vi "add values.vi"(4 "name":string, 5 "index string":string, 6 "is attribute?":bool, 7 "is array element?":bool, 8 "error in (no error)":errorcluster, 9 "Item Indent":i32, 10 "Variant":variant, 11 "Items in":T1(array[cluster])) -> (0 "error out":errorcluster, 3 "Items out":T1(array[cluster]))   [LabVIEW 2016]
uses:
  get unit string.vi
  <vilib>/Utility/Data Type/Get Numeric Information.vi
  <vilib>/Utility/Data Type/Get Cluster Information.vi
  <vilib>/Utility/LVClass/Get LV Class Name.vi
  <vilib>/Utility/Data Type/Get Fixed-Point Information.vi
  <vilib>/Utility/Data Type/Get Refnum Information.vi
  <vilib>/Utility/Data Type/NI_Data Type.lvlib
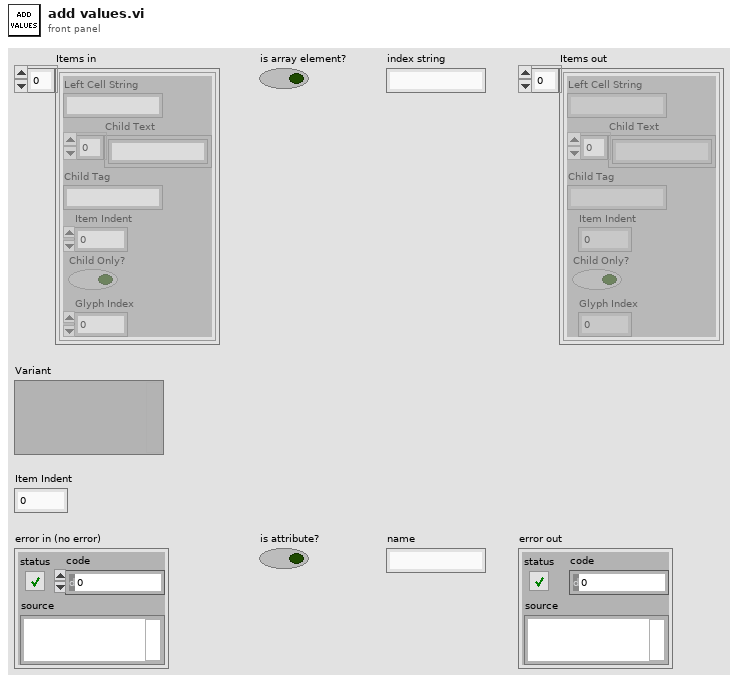
[diagram p1: front panel]
types:
  T1 = cluster{"Left Cell String":string, "Child Text":string[], "Child Tag":string, "Item Indent":i32, "Child Only?":bool, "Glyph Index":i32}[]
  T2 = typedef "NI_Data Type.lvlib/Data Type.ctl" = enum8{"Invalid Type", "Void", "I8", "I16", "I32", "I64", "U8", "U16", "U32", "U64", "Single Float", "Double Float", "Extended Float", "Single Complex", "Double Complex", "Extended Complex", "Enum U8", "Enum U16", "Enum U32", "Enum U64", "Single Float With Unit", "Double Float With Unit", "Extended Float With Unit", "Single Complex with Unit", "Double Complex with Unit", "Extended Complex with Unit", "Boolean", "String", "Path", "Picture", "Tag", "Array", "Cluster", "Variant", "LV Variant", "Waveform", "Timestamp", "Digital Waveform", "Digital Data", "ExpressData", "Refnum", "External Data", "VI", "Poly VI", "LabVIEW Class Instance", "Fixed Point"}
  T3 = cluster{"Left Cell String":string, "Child Text":string[], "Child Tag":string, "Item Indent":i32, "Child Only?":bool, "Glyph Index":i32}
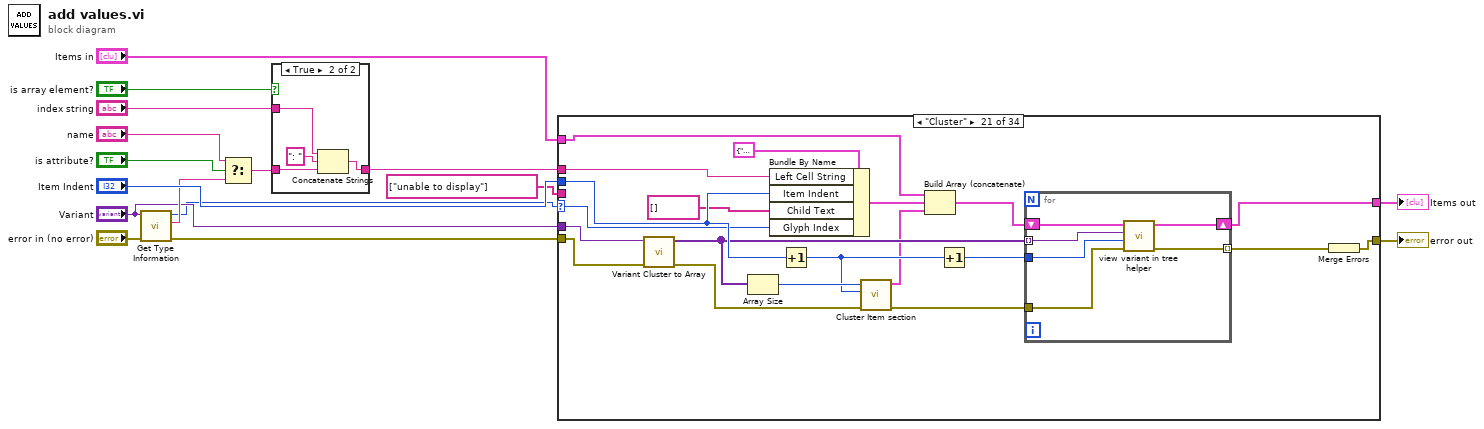
[diagram p0: block diagram]
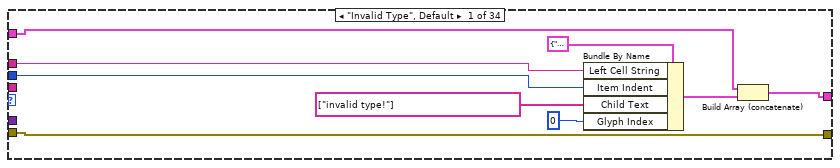
[diagram p3: hidden frame]
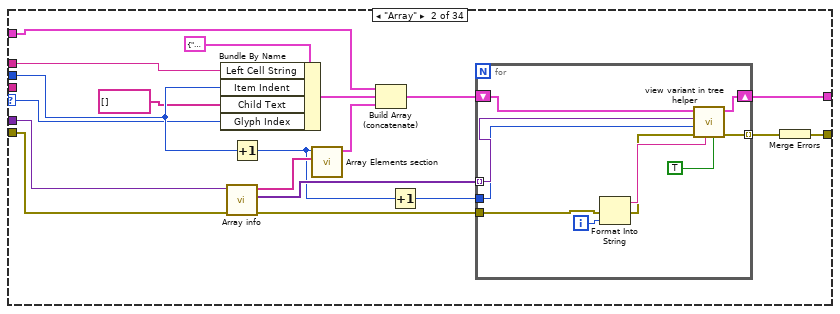
[diagram p4: hidden frame]
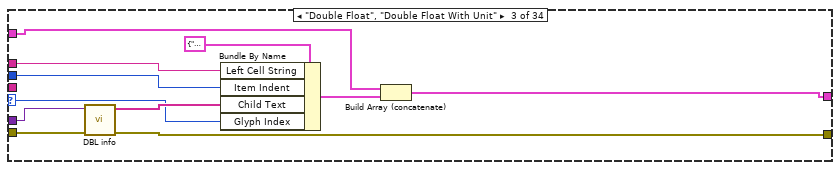
[diagram p5: hidden frame]
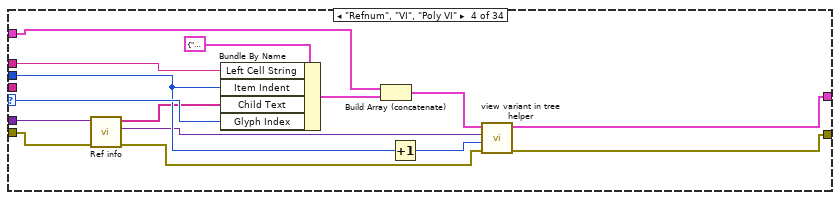
[diagram p6: hidden frame]
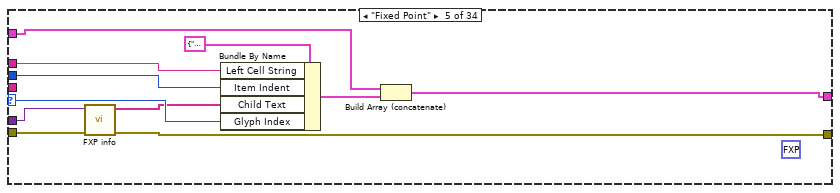
[diagram p7: hidden frame]
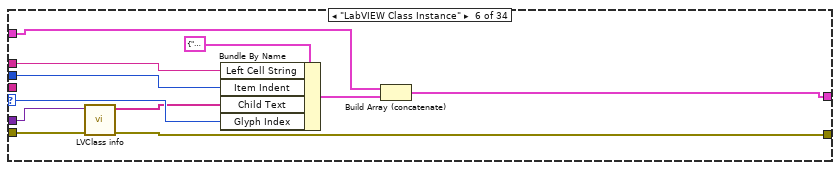
[diagram p8: hidden frame]
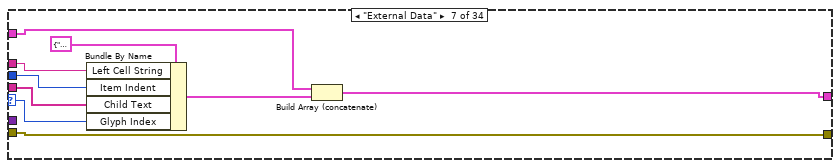
[diagram p9: hidden frame]
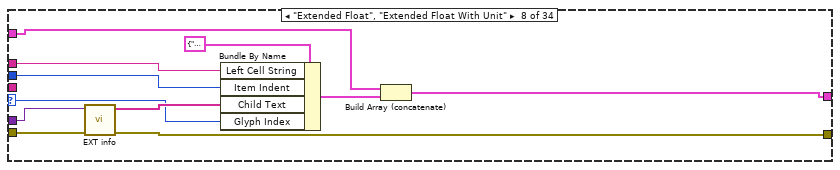
[diagram p10: hidden frame]
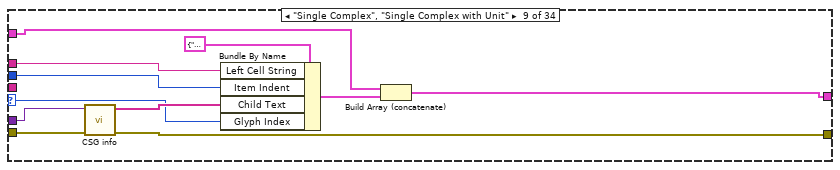
[diagram p11: hidden frame]
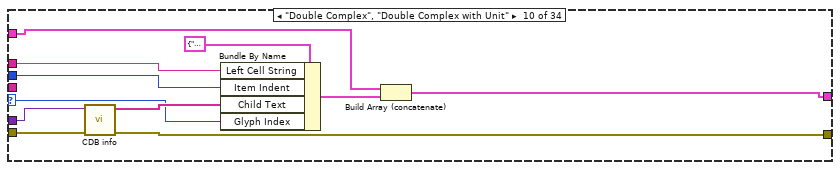
[diagram p12: hidden frame]
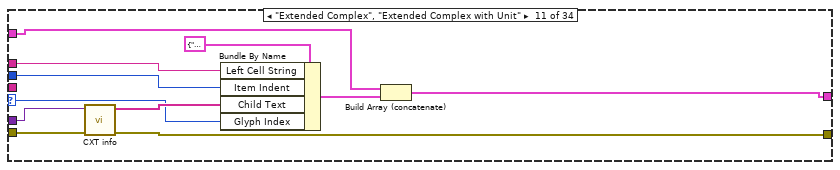
[diagram p13: hidden frame]
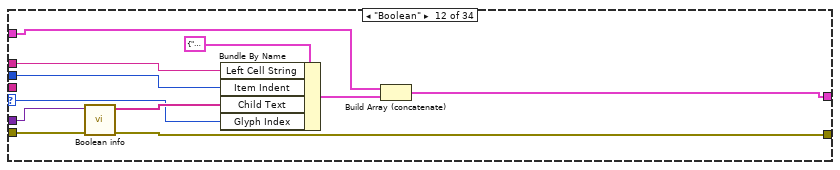
[diagram p14: hidden frame]
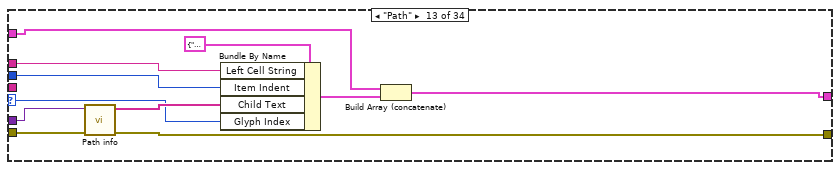
[diagram p15: hidden frame]
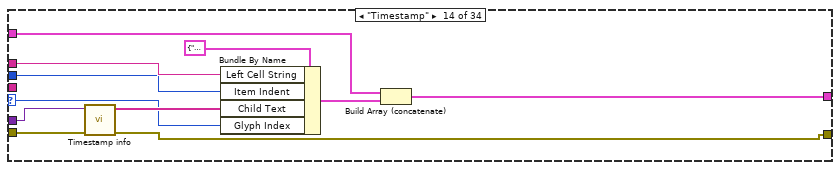
[diagram p16: hidden frame]
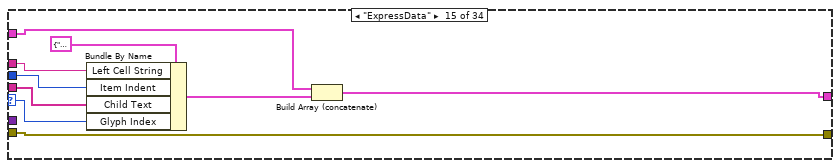
[diagram p17: hidden frame]
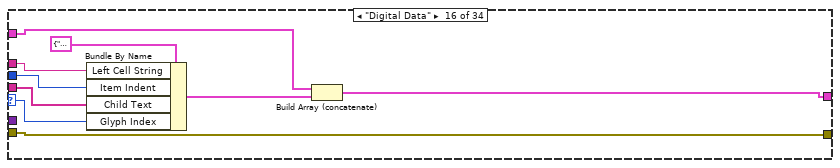
[diagram p18: hidden frame]
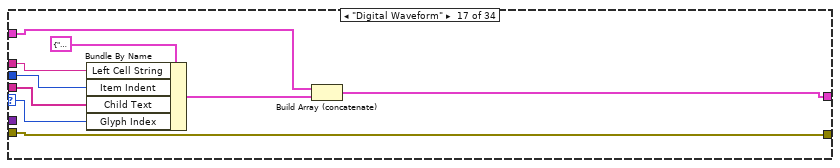
[diagram p19: hidden frame]
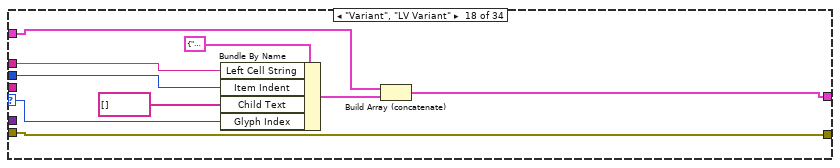
[diagram p20: hidden frame]
diagram:
  n1 = call <vilib>:"Get Type Information.vi"("error in (no error)"="error in (no error)", "Variant"="Variant") -> ("error out"=w15:errorcluster, "Name"=w7:string, "Type"=w1:T2)  [unwired: 5 in, 2 out]
  n2 = Select(t="name", s="is attribute?", f=w7) -> (s? t:f=w12:string)
  n3 = case shown="True" "is array element?" {
    tunnel: "index string" -> [_ w21]
    tunnel: w12 -> [w17 w19]
    tunnel: [w17 w18] -> w13
    frame False {
    }
    frame True {
      n4 = Concatenate Strings(w21, ": " ("string"), w19) -> (w18:string)
    }
  }
  n5 = case shown="\"Cluster\"" w1 {
    selector: w1 -> [_ w39 w64 w82 w90 w101 w110 w120 w131 w142 w153 w163 w174 w185 w195 w204 w213 w223 w232 w240 w257 w275 w284 w294 w305 w317 w327 w338 w349 w360 w371 w382 w393 w404]
    tunnel: "Items in" -> [w25 w46 w67 w80 w93 w104 w113 w123 w134 w145 w156 w166 w177 w188 w199 w208 w217 w227 w236 w244 w265 w279 w288 w297 w310 w321 w332 w343 w354 w365 w376 w387 w398 w409]
    tunnel: "Variant" -> [_ w49 w60 w81 w87 w98 _ w119 w129 w140 w151 w168 w179 w190 _ _ _ _ _ _ w258 _ _ w299 w307 w316 w329 w340 w351 w362 w373 w384 w395 w406]
    tunnel: w13 -> [w22 w40 w61 w84 w95 w106 w115 w126 w137 w148 w159 w170 w181 w192 w201 w210 w219 w228 w237 w246 w266 w281 w290 w301 w312 w323 w334 w345 w356 w367 w378 w389 w400 w411]
    tunnel: "Item Indent" -> [w28 w47 w69 w77 w94 w105 w114 w125 w136 w147 w158 w169 w180 w191 w200 w209 w218 w224 w233 w245 w261 w280 w289 w300 w311 w322 w333 w344 w355 w366 w377 w388 w399 w410]
    tunnel: [w23 w43 w65 w78 w91 w102 w111 w121 w132 w143 w154 w164 w175 w186 w197 w206 w215 w225 w234 w242 w262 w277 w286 w295 w308 w319 w330 w341 w352 w363 w374 w385 w396 w407] -> w5
    tunnel: string[] ["unable to display"] ("Child Text") -> [_ _ _ _ _ _ w108 _ _ _ _ _ _ _ w196 w205 w214 _ _ w241 _ w276 w285 _ _ _ _ _ _ _ _ _ _ _]
    tunnel: w15 -> [w30 w38 w63 w72 w89 w100 w109 w118 w130 w139 w152 w162 w173 w184 w194 w203 w212 w222 w231 w239 w256 w274 w283 w293 w304 w315 w326 w337 w348 w359 w370 w381 w392 w403]
    tunnel: [w30 w35 w62 w75 w88 w99 w109 w117 w128 w141 w150 w161 w172 w183 w194 w203 w212 w222 w231 w239 w252 w274 w283 w292 w303 w314 w325 w336 w347 w358 w369 w380 w391 w402] -> w16
    frame "Invalid Type", Default {
      n6 = Bundle By Name(cluster=T3 {"Left Cell String"="", "Child Text"=[], "Child Tag"="", "Item Indent"=0, "Child Only?"=FALSE, "Glyph Index"=0} ("Item"), "Left Cell String"=w22, "Item Indent"=w28, "Child Text"=string[] ["invalid type!"], "Glyph Index"=0) -> (w24:T3)
      n7 = Build Array (concatenate)(w25, w24) -> (w23:T1)
    }
    frame "Array" {
      n8 = Bundle By Name(cluster=T3 {"Left Cell String"="", "Child Text"=[], "Child Tag"="", "Item Indent"=0, "Child Only?"=FALSE, "Glyph Index"=0} ("Item"), "Left Cell String"=w40, "Item Indent"=w47, "Child Text"=string[] [], "Glyph Index"=w39) -> (w45:T3)
      n9 = call "Array info.vi"("error in (no error)"=w38, "Variant"=w49) -> ("error out"=w37:errorcluster, "elements"=w42:variant[], "child strings"=w41:string[])  [unwired: 7 in]
      n10 = Increment(x=w47) -> (x+1=w34:i32)
      n11 = call "Array Elements section.vi"("child strings"=w41, "indent"=w34) -> ("Array Elements section"=w33:T3)  [unwired: 9 in]
      n12 = Build Array (concatenate)(w46, w45, w33) -> (w44:T1)
      n13 = Increment(x=w34) -> (x+1=w31:i32)
      n14 = for {
        tunnel: w42 -> [w57] mode=indexing
        shift-right: [w58] -> w43
        shift-left: w44 -> [w59]
        tunnel: w31 -> [w56]
        tunnel: w37 -> [w52]
        tunnel: [w50] -> w36 mode=indexing
        i -> [w55]
        n15 = Format Into String(error in=w52, w55) -> (resulting string=w54:string, error out=w51:errorcluster)  [unwired: 2 in]
        n16 = call "view variant in tree helper.vi"("is array element?"=TRUE, "index string"=w54, "error in (no error)"=w51, "Item Indent"=w56, "Variant"=w57, "Items"=w59) -> ("error out"=w50:errorcluster, "Items out"=w58:T1)  [unwired: 4 in]
      }
      n17 = Merge Errors(w36) -> (w35:errorcluster)
    }
    frame "Double Float", "Double Float With Unit" {
      n18 = call "DBL info.vi"("error in (no error)"=w63, "Variant"=w60) -> ("error out"=w62:errorcluster, "child strings"=w68:string[])  [unwired: 8 in]
      n19 = Bundle By Name(cluster=T3 {"Left Cell String"="", "Child Text"=[], "Child Tag"="", "Item Indent"=0, "Child Only?"=FALSE, "Glyph Index"=0} ("Item"), "Left Cell String"=w61, "Item Indent"=w69, "Child Text"=w68, "Glyph Index"=w64) -> (w66:T3)
      n20 = Build Array (concatenate)(w67, w66) -> (w65:T1)
    }
    frame "Refnum", "VI", "Poly VI" {
      n21 = call "Ref info.vi"("error in (no error)"=w72, "Variant"=w81) -> ("error out"=w71:errorcluster, "refnum type"=w73:variant, "child strings"=w74:string[])  [unwired: 7 in]
      n22 = Bundle By Name(cluster=T3 {"Left Cell String"="", "Child Text"=[], "Child Tag"="", "Item Indent"=0, "Child Only?"=FALSE, "Glyph Index"=0} ("Item"), "Left Cell String"=w84, "Item Indent"=w77, "Child Text"=w74, "Glyph Index"=w82) -> (w83:T3)
      n23 = Build Array (concatenate)(w80, w83) -> (w79:T1)
      n24 = Increment(x=w77) -> (x+1=w76:i32)
      n25 = call "view variant in tree helper.vi"("error in (no error)"=w71, "Item Indent"=w76, "Variant"=w73, "Items"=w79) -> ("error out"=w75:errorcluster, "Items out"=w78:T1)  [unwired: 6 in]
    }
    frame "Fixed Point" {
      (unwired) fxp<+,1,1> 0.0
      n26 = call "FXP info.vi"("error in (no error)"=w89, "Variant"=w87) -> ("error out"=w88:errorcluster, "child strings"=w86:string[])  [unwired: 8 in]
      n27 = Bundle By Name(cluster=T3 {"Left Cell String"="", "Child Text"=[], "Child Tag"="", "Item Indent"=0, "Child Only?"=FALSE, "Glyph Index"=0} ("Item"), "Left Cell String"=w95, "Item Indent"=w94, "Child Text"=w86, "Glyph Index"=w90) -> (w92:T3)
      n28 = Build Array (concatenate)(w93, w92) -> (w91:T1)
    }
    frame "LabVIEW Class Instance" {
      n29 = call "LVClass info.vi"("error in (no error)"=w100, "Variant"=w98) -> ("error out"=w99:errorcluster, "child strings"=w97:string[])  [unwired: 8 in]
      n30 = Bundle By Name(cluster=T3 {"Left Cell String"="", "Child Text"=[], "Child Tag"="", "Item Indent"=0, "Child Only?"=FALSE, "Glyph Index"=0} ("Item"), "Left Cell String"=w106, "Item Indent"=w105, "Child Text"=w97, "Glyph Index"=w101) -> (w103:T3)
      n31 = Build Array (concatenate)(w104, w103) -> (w102:T1)
    }
    frame "External Data" {
      n32 = Bundle By Name(cluster=T3 {"Left Cell String"="", "Child Text"=[], "Child Tag"="", "Item Indent"=0, "Child Only?"=FALSE, "Glyph Index"=0} ("Item"), "Left Cell String"=w115, "Item Indent"=w114, "Child Text"=w108, "Glyph Index"=w110) -> (w112:T3)
      n33 = Build Array (concatenate)(w113, w112) -> (w111:T1)
    }
    frame "Extended Float", "Extended Float With Unit" {
      n34 = call "EXT info.vi"("error in (no error)"=w118, "Variant"=w119) -> ("error out"=w117:errorcluster, "child strings"=w124:string[])  [unwired: 8 in]
      n35 = Bundle By Name(cluster=T3 {"Left Cell String"="", "Child Text"=[], "Child Tag"="", "Item Indent"=0, "Child Only?"=FALSE, "Glyph Index"=0} ("Item"), "Left Cell String"=w126, "Item Indent"=w125, "Child Text"=w124, "Glyph Index"=w120) -> (w122:T3)
      n36 = Build Array (concatenate)(w123, w122) -> (w121:T1)
    }
    frame "Single Complex", "Single Complex with Unit" {
      n37 = call "CSG info.vi"("error in (no error)"=w130, "Variant"=w129) -> ("error out"=w128:errorcluster, "child strings"=w135:string[])  [unwired: 8 in]
      n38 = Bundle By Name(cluster=T3 {"Left Cell String"="", "Child Text"=[], "Child Tag"="", "Item Indent"=0, "Child Only?"=FALSE, "Glyph Index"=0} ("Item"), "Left Cell String"=w137, "Item Indent"=w136, "Child Text"=w135, "Glyph Index"=w131) -> (w133:T3)
      n39 = Build Array (concatenate)(w134, w133) -> (w132:T1)
    }
    frame "Double Complex", "Double Complex with Unit" {
      n40 = call "CDB info.vi"("error in (no error)"=w139, "Variant"=w140) -> ("error out"=w141:errorcluster, "child strings"=w146:string[])  [unwired: 8 in]
      n41 = Bundle By Name(cluster=T3 {"Left Cell String"="", "Child Text"=[], "Child Tag"="", "Item Indent"=0, "Child Only?"=FALSE, "Glyph Index"=0} ("Item"), "Left Cell String"=w148, "Item Indent"=w147, "Child Text"=w146, "Glyph Index"=w142) -> (w144:T3)
      n42 = Build Array (concatenate)(w145, w144) -> (w143:T1)
    }
    frame "Extended Complex", "Extended Complex with Unit" {
      n43 = call "CXT info.vi"("error in (no error)"=w152, "Variant"=w151) -> ("error out"=w150:errorcluster, "child strings"=w157:string[])  [unwired: 8 in]
      n44 = Bundle By Name(cluster=T3 {"Left Cell String"="", "Child Text"=[], "Child Tag"="", "Item Indent"=0, "Child Only?"=FALSE, "Glyph Index"=0} ("Item"), "Left Cell String"=w159, "Item Indent"=w158, "Child Text"=w157, "Glyph Index"=w153) -> (w155:T3)
      n45 = Build Array (concatenate)(w156, w155) -> (w154:T1)
    }
    frame "Boolean" {
      n46 = call "Boolean info.vi"("error in (no error)"=w162, "Variant"=w168) -> ("error out"=w161:errorcluster, "child strings"=w167:string[])  [unwired: 8 in]
      n47 = Bundle By Name(cluster=T3 {"Left Cell String"="", "Child Text"=[], "Child Tag"="", "Item Indent"=0, "Child Only?"=FALSE, "Glyph Index"=0} ("Item"), "Left Cell String"=w170, "Item Indent"=w169, "Child Text"=w167, "Glyph Index"=w163) -> (w165:T3)
      n48 = Build Array (concatenate)(w166, w165) -> (w164:T1)
    }
    frame "Path" {
      n49 = call "Path info.vi"("error in (no error)"=w173, "Variant"=w179) -> ("error out"=w172:errorcluster, "child strings"=w178:string[])  [unwired: 8 in]
      n50 = Bundle By Name(cluster=T3 {"Left Cell String"="", "Child Text"=[], "Child Tag"="", "Item Indent"=0, "Child Only?"=FALSE, "Glyph Index"=0} ("Item"), "Left Cell String"=w181, "Item Indent"=w180, "Child Text"=w178, "Glyph Index"=w174) -> (w176:T3)
      n51 = Build Array (concatenate)(w177, w176) -> (w175:T1)
    }
    frame "Timestamp" {
      n52 = call "Timestamp info.vi"("error in (no error)"=w184, "Variant"=w190) -> ("error out"=w183:errorcluster, "child strings"=w189:string[])  [unwired: 8 in]
      n53 = Bundle By Name(cluster=T3 {"Left Cell String"="", "Child Text"=[], "Child Tag"="", "Item Indent"=0, "Child Only?"=FALSE, "Glyph Index"=0} ("Item"), "Left Cell String"=w192, "Item Indent"=w191, "Child Text"=w189, "Glyph Index"=w185) -> (w187:T3)
      n54 = Build Array (concatenate)(w188, w187) -> (w186:T1)
    }
    frame "ExpressData" {
      n55 = Bundle By Name(cluster=T3 {"Left Cell String"="", "Child Text"=[], "Child Tag"="", "Item Indent"=0, "Child Only?"=FALSE, "Glyph Index"=0} ("Item"), "Left Cell String"=w201, "Item Indent"=w200, "Child Text"=w196, "Glyph Index"=w195) -> (w198:T3)
      n56 = Build Array (concatenate)(w199, w198) -> (w197:T1)
    }
    frame "Digital Data" {
      n57 = Bundle By Name(cluster=T3 {"Left Cell String"="", "Child Text"=[], "Child Tag"="", "Item Indent"=0, "Child Only?"=FALSE, "Glyph Index"=0} ("Item"), "Left Cell String"=w210, "Item Indent"=w209, "Child Text"=w205, "Glyph Index"=w204) -> (w207:T3)
      n58 = Build Array (concatenate)(w208, w207) -> (w206:T1)
    }
    frame "Digital Waveform" {
      n59 = Bundle By Name(cluster=T3 {"Left Cell String"="", "Child Text"=[], "Child Tag"="", "Item Indent"=0, "Child Only?"=FALSE, "Glyph Index"=0} ("Item"), "Left Cell String"=w219, "Item Indent"=w218, "Child Text"=w214, "Glyph Index"=w213) -> (w216:T3)
      n60 = Build Array (concatenate)(w217, w216) -> (w215:T1)
    }
    frame "Variant", "LV Variant" {
      n61 = Bundle By Name(cluster=T3 {"Left Cell String"="", "Child Text"=[], "Child Tag"="", "Item Indent"=0, "Child Only?"=FALSE, "Glyph Index"=0} ("Item"), "Left Cell String"=w228, "Item Indent"=w224, "Child Text"=string[] [], "Glyph Index"=w223) -> (w226:T3)
      n62 = Build Array (concatenate)(w227, w226) -> (w225:T1)
    }
    frame "Void" {
      n63 = Bundle By Name(cluster=T3 {"Left Cell String"="", "Child Text"=[], "Child Tag"="", "Item Indent"=0, "Child Only?"=FALSE, "Glyph Index"=0} ("Item"), "Left Cell String"=w237, "Item Indent"=w233, "Child Text"=string[] ["<void>"], "Glyph Index"=w232) -> (w235:T3)
      n64 = Build Array (concatenate)(w236, w235) -> (w234:T1)
    }
    frame "Waveform" {
      n65 = Bundle By Name(cluster=T3 {"Left Cell String"="", "Child Text"=[], "Child Tag"="", "Item Indent"=0, "Child Only?"=FALSE, "Glyph Index"=0} ("Item"), "Left Cell String"=w246, "Item Indent"=w245, "Child Text"=w241, "Glyph Index"=w240) -> (w243:T3)
      n66 = Build Array (concatenate)(w244, w243) -> (w242:T1)
    }
    frame "Cluster" {
      n67 = call "Variant Cluster to Array.vi"("error in (no error)"=w256, "Cluster"=w258) -> ("error out"=w255:errorcluster, "Array"=w260:variant[])  [unwired: 8 in]
      n68 = Array Size(array=w260) -> (size(s)=w259:i32)
      n69 = Bundle By Name(cluster=T3 {"Left Cell String"="", "Child Text"=[], "Child Tag"="", "Item Indent"=0, "Child Only?"=FALSE, "Glyph Index"=0} ("Item"), "Left Cell String"=w266, "Item Indent"=w261, "Child Text"=string[] [], "Glyph Index"=w257) -> (w264:T3)
      n70 = Increment(x=w261) -> (x+1=w251:i32)
      n71 = call "Cluster Item section.vi"("error in (no error)"=w255, "indent"=w251, "count"=w259) -> ("error out"=w254:errorcluster, "Cluster Item"=w249:T3)  [unwired: 7 in]
      n72 = Build Array (concatenate)(w265, w264, w249) -> (w263:T1)
      n73 = Increment(x=w251) -> (x+1=w248:i32)
      n74 = for {
        tunnel: w260 -> [w272] mode=indexing
        shift-right: [w271] -> w262
        shift-left: w263 -> [w273]
        tunnel: w248 -> [w270]
        tunnel: w254 -> [w269]
        tunnel: [w268] -> w253 mode=indexing
        n75 = call "view variant in tree helper.vi"("error in (no error)"=w269, "Item Indent"=w270, "Variant"=w272, "Items"=w273) -> ("error out"=w268:errorcluster, "Items out"=w271:T1)  [unwired: 6 in]
      }
      n76 = Merge Errors(w253) -> (w252:errorcluster)
    }
    frame "Tag" {
      n77 = Bundle By Name(cluster=T3 {"Left Cell String"="", "Child Text"=[], "Child Tag"="", "Item Indent"=0, "Child Only?"=FALSE, "Glyph Index"=0} ("Item"), "Left Cell String"=w281, "Item Indent"=w280, "Child Text"=w276, "Glyph Index"=w275) -> (w278:T3)
      n78 = Build Array (concatenate)(w279, w278) -> (w277:T1)
    }
    frame "Picture" {
      n79 = Bundle By Name(cluster=T3 {"Left Cell String"="", "Child Text"=[], "Child Tag"="", "Item Indent"=0, "Child Only?"=FALSE, "Glyph Index"=0} ("Item"), "Left Cell String"=w290, "Item Indent"=w289, "Child Text"=w285, "Glyph Index"=w284) -> (w287:T3)
      n80 = Build Array (concatenate)(w288, w287) -> (w286:T1)
    }
    frame "String" {
      n81 = call "String info.vi"("error in (no error)"=w293, "Variant"=w299) -> ("error out"=w292:errorcluster, "child strings"=w298:string[])  [unwired: 8 in]
      n82 = Bundle By Name(cluster=T3 {"Left Cell String"="", "Child Text"=[], "Child Tag"="", "Item Indent"=0, "Child Only?"=FALSE, "Glyph Index"=0} ("Item"), "Left Cell String"=w301, "Item Indent"=w300, "Child Text"=w298, "Glyph Index"=w294) -> (w296:T3)
      n83 = Build Array (concatenate)(w297, w296) -> (w295:T1)
    }
    frame "Enum U8".."Enum U64" {
      n84 = call "Enum info.vi"("error in (no error)"=w304, "Variant"=w307) -> ("error out"=w303:errorcluster, "child strings"=w306:string[])  [unwired: 8 in]
      n85 = Bundle By Name(cluster=T3 {"Left Cell String"="", "Child Text"=[], "Child Tag"="", "Item Indent"=0, "Child Only?"=FALSE, "Glyph Index"=0} ("Item"), "Left Cell String"=w312, "Item Indent"=w311, "Child Text"=w306, "Glyph Index"=w305) -> (w309:T3)
      n86 = Build Array (concatenate)(w310, w309) -> (w308:T1)
    }
    frame "Single Float", "Single Float With Unit" {
      n87 = call "SGL info.vi"("error in (no error)"=w315, "Variant"=w316) -> ("error out"=w314:errorcluster, "child strings"=w318:string[])  [unwired: 8 in]
      n88 = Bundle By Name(cluster=T3 {"Left Cell String"="", "Child Text"=[], "Child Tag"="", "Item Indent"=0, "Child Only?"=FALSE, "Glyph Index"=0} ("Item"), "Left Cell String"=w323, "Item Indent"=w322, "Child Text"=w318, "Glyph Index"=w317) -> (w320:T3)
      n89 = Build Array (concatenate)(w321, w320) -> (w319:T1)
    }
    frame "I8" {
      n90 = call "I8 info.vi"("error in (no error)"=w326, "Variant"=w329) -> ("error out"=w325:errorcluster, "child strings"=w328:string[])  [unwired: 8 in]
      n91 = Bundle By Name(cluster=T3 {"Left Cell String"="", "Child Text"=[], "Child Tag"="", "Item Indent"=0, "Child Only?"=FALSE, "Glyph Index"=0} ("Item"), "Left Cell String"=w334, "Item Indent"=w333, "Child Text"=w328, "Glyph Index"=w327) -> (w331:T3)
      n92 = Build Array (concatenate)(w332, w331) -> (w330:T1)
    }
    frame "I16" {
      n93 = call "I16 info.vi"("error in (no error)"=w337, "Variant"=w340) -> ("error out"=w336:errorcluster, "child strings"=w339:string[])  [unwired: 8 in]
      n94 = Bundle By Name(cluster=T3 {"Left Cell String"="", "Child Text"=[], "Child Tag"="", "Item Indent"=0, "Child Only?"=FALSE, "Glyph Index"=0} ("Item"), "Left Cell String"=w345, "Item Indent"=w344, "Child Text"=w339, "Glyph Index"=w338) -> (w342:T3)
      n95 = Build Array (concatenate)(w343, w342) -> (w341:T1)
    }
    frame "I32" {
      n96 = call "I32.vi"("error in (no error)"=w348, "Variant"=w351) -> ("error out"=w347:errorcluster, "child strings"=w350:string[])  [unwired: 8 in]
      n97 = Bundle By Name(cluster=T3 {"Left Cell String"="", "Child Text"=[], "Child Tag"="", "Item Indent"=0, "Child Only?"=FALSE, "Glyph Index"=0} ("Item"), "Left Cell String"=w356, "Item Indent"=w355, "Child Text"=w350, "Glyph Index"=w349) -> (w353:T3)
      n98 = Build Array (concatenate)(w354, w353) -> (w352:T1)
    }
    frame "I64" {
      n99 = call "I64 info.vi"("error in (no error)"=w359, "Variant"=w362) -> ("error out"=w358:errorcluster, "child strings"=w361:string[])  [unwired: 8 in]
      n100 = Bundle By Name(cluster=T3 {"Left Cell String"="", "Child Text"=[], "Child Tag"="", "Item Indent"=0, "Child Only?"=FALSE, "Glyph Index"=0} ("Item"), "Left Cell String"=w367, "Item Indent"=w366, "Child Text"=w361, "Glyph Index"=w360) -> (w364:T3)
      n101 = Build Array (concatenate)(w365, w364) -> (w363:T1)
    }
    frame "U8" {
      n102 = call "U8 info.vi"("error in (no error)"=w370, "Variant"=w373) -> ("error out"=w369:errorcluster, "child strings"=w372:string[])  [unwired: 8 in]
      n103 = Bundle By Name(cluster=T3 {"Left Cell String"="", "Child Text"=[], "Child Tag"="", "Item Indent"=0, "Child Only?"=FALSE, "Glyph Index"=0} ("Item"), "Left Cell String"=w378, "Item Indent"=w377, "Child Text"=w372, "Glyph Index"=w371) -> (w375:T3)
      n104 = Build Array (concatenate)(w376, w375) -> (w374:T1)
    }
    frame "U16" {
      n105 = call "U16 info.vi"("error in (no error)"=w381, "Variant"=w384) -> ("error out"=w380:errorcluster, "child strings"=w383:string[])  [unwired: 8 in]
      n106 = Bundle By Name(cluster=T3 {"Left Cell String"="", "Child Text"=[], "Child Tag"="", "Item Indent"=0, "Child Only?"=FALSE, "Glyph Index"=0} ("Item"), "Left Cell String"=w389, "Item Indent"=w388, "Child Text"=w383, "Glyph Index"=w382) -> (w386:T3)
      n107 = Build Array (concatenate)(w387, w386) -> (w385:T1)
    }
    frame "U32" {
      n108 = call "U32 info.vi"("error in (no error)"=w392, "Variant"=w395) -> ("error out"=w391:errorcluster, "child strings"=w394:string[])  [unwired: 8 in]
      n109 = Bundle By Name(cluster=T3 {"Left Cell String"="", "Child Text"=[], "Child Tag"="", "Item Indent"=0, "Child Only?"=FALSE, "Glyph Index"=0} ("Item"), "Left Cell String"=w400, "Item Indent"=w399, "Child Text"=w394, "Glyph Index"=w393) -> (w397:T3)
      n110 = Build Array (concatenate)(w398, w397) -> (w396:T1)
    }
    frame "U64" {
      n111 = call "U64 info.vi"("error in (no error)"=w403, "Variant"=w406) -> ("error out"=w402:errorcluster, "child strings"=w405:string[])  [unwired: 8 in]
      n112 = Bundle By Name(cluster=T3 {"Left Cell String"="", "Child Text"=[], "Child Tag"="", "Item Indent"=0, "Child Only?"=FALSE, "Glyph Index"=0} ("Item"), "Left Cell String"=w411, "Item Indent"=w410, "Child Text"=w405, "Glyph Index"=w404) -> (w408:T3)
      n113 = Build Array (concatenate)(w409, w408) -> (w407:T1)
    }
  }
  "error out" <- w16
  "Items out" <- w5
